vi "Prepare.vi"(8 "Error In":errorcluster) -> (0 "Error Out":errorcluster)   [LabVIEW 2019]
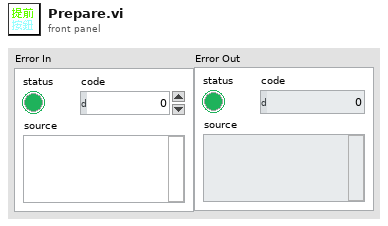
[diagram p1: front panel]
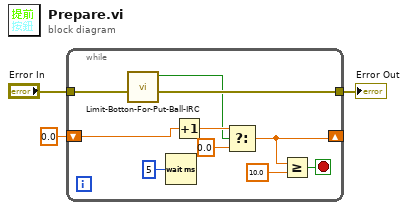
[diagram p0: block diagram]
diagram:
  n1 = while {
    tunnel: "Error In" -> [w5]
    tunnel: [w6] -> w2
    shift-right: [w8] -> _
    shift-left: 0.0 ("f") -> [w11]
    stop <- w9 stop-if-true
    n2 = call "Limit-Botton-For-Put-Ball-IRC.vi"("Error In"=w5) -> ("Error Out"=w6:errorcluster, "放球校正微動觸發?"=w4:bool)  [unwired: 9 in]
    n3 = Wait (ms)(milliseconds to wait=u32 5) -> ()  [unwired: 1 out]
    n4 = Increment(x=w11) -> (x+1=w12:dbl)
    n5 = Select(t=w12, s=w4, f=0.0) -> (s? t:f=w8:dbl)
    n6 = Greater Or Equal?(x=w8, y=10.0) -> (x >= y?=w9:bool)
  }
  "Error Out" <- w2
